vi "add_elementToAgents.vi"(0 "Host_Reference":refnum<class "HGF_Reference.lvclass">, 2 "timeout in ms (-1)":i32=-1, 3 "Agent ID":string, 5 "error in (no error)":errorcluster) -> (14 "dup Host_Reference":refnum<class "HGF_Reference.lvclass">, 17 "empty ID":bool, 19 "error out":errorcluster)   [LabVIEW 2009, in "MoAgSy.lvlib" / "MoAgSy_Host.lvclass"]
doc: "<B>public</B> VI adds an Agents ID to the Hosts running agents list.\nIs called by add agent vi.\n\nF.Berck@gsi.de\nGSI Darmstadt 2009"
uses:
  MoAgSy_Host.lvclass
  HGF_BaseClasses/HGF_Reference/HGF_Reference.lvclass
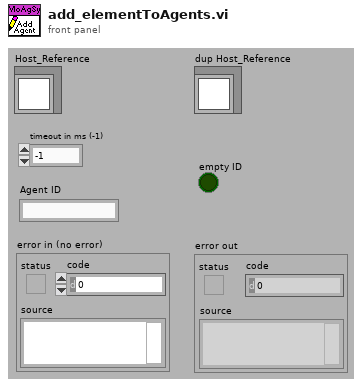
[diagram p1: front panel]
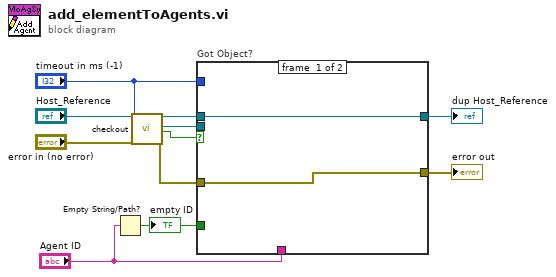
[diagram p0: block diagram]
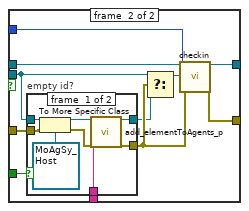
[diagram p2: hidden frame]
diagram:
  n1 = Empty String/Path?(string/path="Agent ID") -> (empty?=w1:bool)
  "empty ID" <- w1
  n2 = call "checkout.vi"("HGF_Reference"="Host_Reference", "timeout in ms (-1)"="timeout in ms (-1)", "error in (no error)"="error in (no error)") -> ("dup HGF_Reference"=w9:refnum<class "HGF_Reference.lvclass">, "Object"=w10:refnum<class>, "got object?"=w2:bool, "error out"=w11:errorcluster)  [unwired: 13 out]
  n3 = case "Got Object?" shown="True" w2 {
    tunnel: w10 -> [_ w19]
    tunnel: w9 -> [w13 w24]
    tunnel: [w13 w23] -> w5
    tunnel: "timeout in ms (-1)" -> [_ w22]
    tunnel: [w12 w21] -> w6
    tunnel: w11 -> [w12 w20]
    tunnel: "Agent ID" -> [_ w15]
    tunnel: w1 -> [_ w14]
    frame #0 {
    }
    frame #1 {
      n4 = case "empty id?" shown="False" w14 {
        tunnel: w20 -> [w31 w33]
        tunnel: w19 -> [w30 w34]
        tunnel: [w27 w33] -> w17
        tunnel: [w26 w34] -> w16
        tunnel: w15 -> [w25 _]
        frame #0 {
          n5 = To More Specific Class(target class=refnum<class "MoAgSy_Host.lvclass"> refnum ("MoAgSy.lvlib:MoAgSy_Host.lvclass"), reference=w30, error in=w31) -> (specific class reference=w29:refnum<class "MoAgSy_Host.lvclass">, error out=w28:errorcluster)
          n6 = call "add_elementToAgents_p.vi"("MoAgSy_Host"=w29, "Agent ID"=w25, "error in (no error)"=w28) -> ("dup MoAgSy_Host"=w26:refnum<class "MoAgSy_Host.lvclass">, "error out"=w27:errorcluster)  [unwired: 15 out]
        }
        frame #1 {
        }
      }
      n7 = Select(t=w19, s=w17, f=w16) -> (s? t:f=w18:refnum<class>)
      n8 = call "checkin.vi"("HGF_Reference"=w24, "Object"=w18, "timeout /ms (-1)"=w22, "error in (no error)"=w17) -> ("dup HGF_Reference"=w23:refnum<class "HGF_Reference.lvclass">, "error out"=w21:errorcluster)  [unwired: 14 out]
    }
  }
  "dup Host_Reference" <- w5
  "error out" <- w6
